vi "XYdata remove duplicates.vi"(5 "Remove duplicate":bool, 6 "tolerance":dbl=0.0005 format="%.3e", 7 "ascending":bool, 9 "Sort?":bool, 11 "2D input":dbl[][](array[numeric])) -> (3 "2D output":dbl[][](array[numeric]))   [LabVIEW 2019]
panel:
  out "comparative":dbl
  # "(1) Data are sorted ascending or descending order.\n(2) Remove duplicate\n      i) Neighboring two data points are compared, if determined to be a duplicate, the second data point will be removed.\n      ii) Repeat i) unitl no duplicates found."
  # "Caution: All rows will be affected."
  # "(1) Select datasets to be processed"
  # "(2) Sort"
  # "i) Sort ?"
  # "ii) Ascending or descendingwhich order?"
  # "descending"
  # "(3) Remove duplicate? Tolerance?"
  # "(duplicate if \ndata difference <= (max-min) * tolerance"
  # "(4) Start processing"
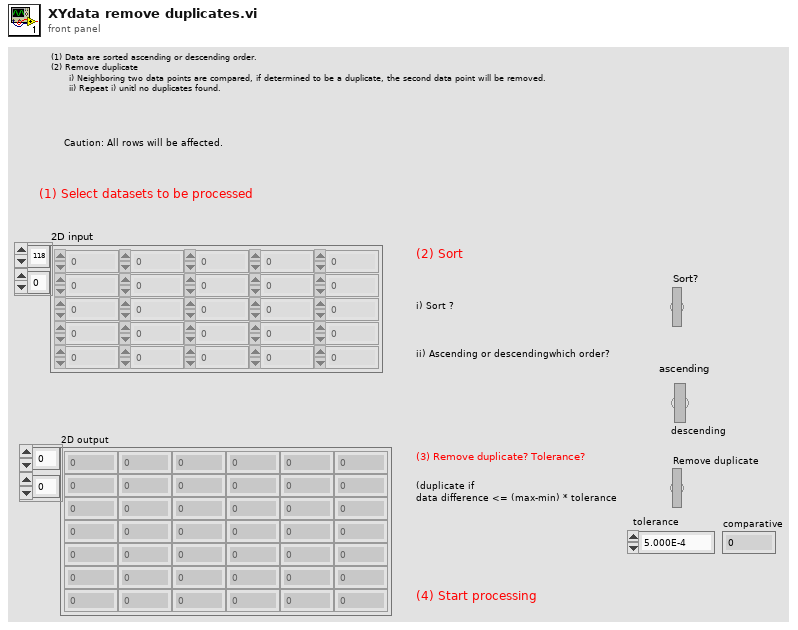
[diagram p1: front panel]
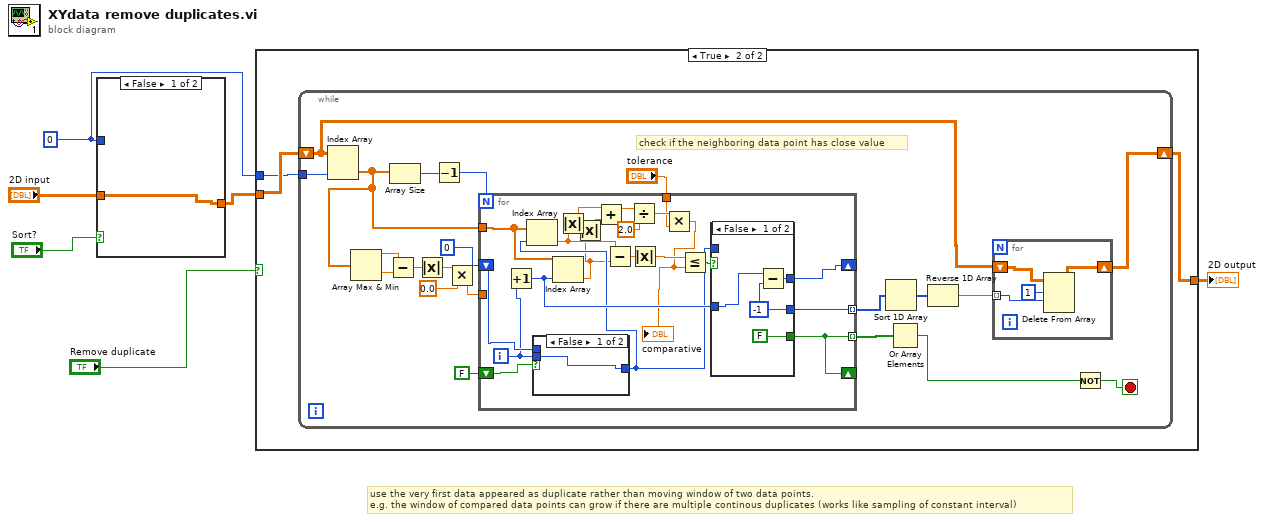
[diagram p0: block diagram]
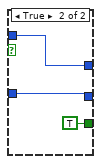
[diagram p4: hidden frame]
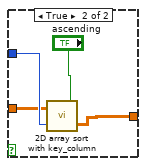
[diagram p5: hidden frame]
diagram:
  w3 = u16 0 ("target column")
  # "use the very first data appeared as duplicate rather than moving window of two data points.\ne.g. the window of compared data points can grow if there are multiple continous duplicates (works like sampling of constant interval)"
  n1 = case shown="False" "Sort?" {
    tunnel: [w7 w11] -> w5
    tunnel: w3 -> [_ w9]
    tunnel: "2D input" -> [w7 w8]
    frame False {
    }
    frame True {
      n2 = call "2D array sort with key_column.vi"("ascending"="ascending", "key column"=w9, "input"=w8) -> ("output"=w11:dbl[][])
    }
  }
  n3 = case shown="True" "Remove duplicate" {
    tunnel: [w12 w13] -> w1
    tunnel: w5 -> [w12 w15]
    tunnel: w3 -> [_ w14]
    frame False {
    }
    frame True {
      n4 = while {
        tunnel: w14 -> [w30]
        shift-right: [w22] -> w13
        shift-left: w15 -> [w23]
        stop <- w31 stop-if-true
        # "check if the neighboring data point has close value"
        n5 = Index Array(array=w23, index (col)=w30) -> (element=w26:dbl[])  [unwired: 1 in]
        n6 = Array Max & Min(array=w26) -> (max value=w25:dbl, min value=w27:dbl)  [unwired: 2 out]
        n7 = Subtract(x=w25, y=w27) -> (x-y=w28:dbl)
        n8 = Array Size(array=w26) -> (size(s)=w21:i32)
        n9 = Absolute Value(x=w28) -> (abs(x)=w29:dbl)
        n10 = Decrement(x=w21) -> (x-1=w20:i32)
        n11 = Multiply(x=w29, y=0.0) -> (x*y=w24:dbl)
        n12 = for {
          N: w20 -> [_]
          tunnel: w26 -> [w61]
          tunnel: w24 -> [_]
          tunnel: [w55] -> w35 mode=indexing
          tunnel: [w56] -> w33 mode=indexing
          shift-right: [w54] -> _
          shift-left: 0 -> [w52]
          shift-right: [w56] -> _
          shift-left: FALSE -> [w53]
          tunnel: "tolerance" -> [w42]
          i -> [w50]
          n13 = Increment(x=w50) -> (x+1=w58:i32)
          n14 = case shown="False" w53 {
            tunnel: [w62 w63] -> w51
            tunnel: w52 -> [_ w63]
            tunnel: w50 -> [w62 _]
            frame False {
            }
            frame True {
            }
          }
          n15 = Index Array(array=w61, index=w51) -> (element=w49:dbl)
          n16 = Index Array(array=w61, index=w58) -> (element=w48:dbl)
          n17 = Absolute Value(x=w49) -> (abs(x)=w44:dbl)
          n18 = Absolute Value(x=w48) -> (abs(x)=w43:dbl)
          n19 = Add(x=w44, y=w43) -> (x+y=w47:dbl)
          n20 = Subtract(x=w49, y=w48) -> (x-y=w60:dbl)
          n21 = Divide(x=w47, y=2.0) -> (x/y=w45:dbl)
          n22 = Absolute Value(x=w60) -> (abs(x)=w57:dbl)
          n23 = Multiply(x=w45, y=w42) -> (x*y=w41:dbl)
          "comparative" <- w41
          n24 = Less Or Equal?(x=w57, y=w41) -> (x <= y?=w59:bool)
          n25 = case shown="False" w59 {
            tunnel: w58 -> [w65 w70]
            tunnel: [w66 w70] -> w55
            tunnel: [FALSE TRUE] -> w56
            tunnel: [w64 w68] -> w54
            tunnel: w51 -> [_ w68]
            frame False {
              w66 = -1
              n26 = Subtract(x=w65, y=w66) -> (x-y=w64:i32)
            }
            frame True {
            }
          }
        }
        n27 = Sort 1D Array(array=w35) -> (sorted array=w36:i32[])
        n28 = Or Array Elements(Boolean array=w33) -> (logical OR=w32:bool)
        n29 = Reverse 1D Array(array=w36) -> (reversed array=w34:i32[])
        n30 = for {
          tunnel: w34 -> [w39] mode=indexing
          shift-right: [w37] -> w22
          shift-left: w23 -> [w38]
          n31 = Delete From Array(array=w38, length=1, index (row)=w39) -> (array with subset deleted=w37:dbl[][])  [unwired: 1 in, 1 out]
        }
        n32 = Not(x=w32) -> (.not. x?=w31:bool)
      }
    }
  }
  "2D output" <- w1
